vi "600 rpm peristaltic pump multiple heads (mLpermin).vi"(4 "State":i16, 5 "Time":dbl format="%.2f", 6 "Sensor Values":dbl[](array[numeric]), 7 "Set Points":dbl[](array[numeric])) -> (0 "required data":T1={"Set Point names"=["flow rate (mL/min)", "Tubing size code", "# of pump heads"], "required number of setpoints"=3, "required number of sensors"=0, "Sensor names"=[]}, 3 "output value":dbl)   [LabVIEW 2012]
panel:
  in  "pumpflow":dbl[unit][](array[numeric])=[9.549296547316535e-09, 3.342253804929783e-08, 1.2732395447351617e-07, 2.705634032562094e-07, 4.4563384065730255e-07, 6.04788783748884e-07] format="%.3f"
  in  "tubing size":enum16{"13", "14", "16", "25", "17", "18"}(ring)
  # "Enter the correct information for this control code in the required data structure below. Then make the current value default by right clicking on the border of the data structure."
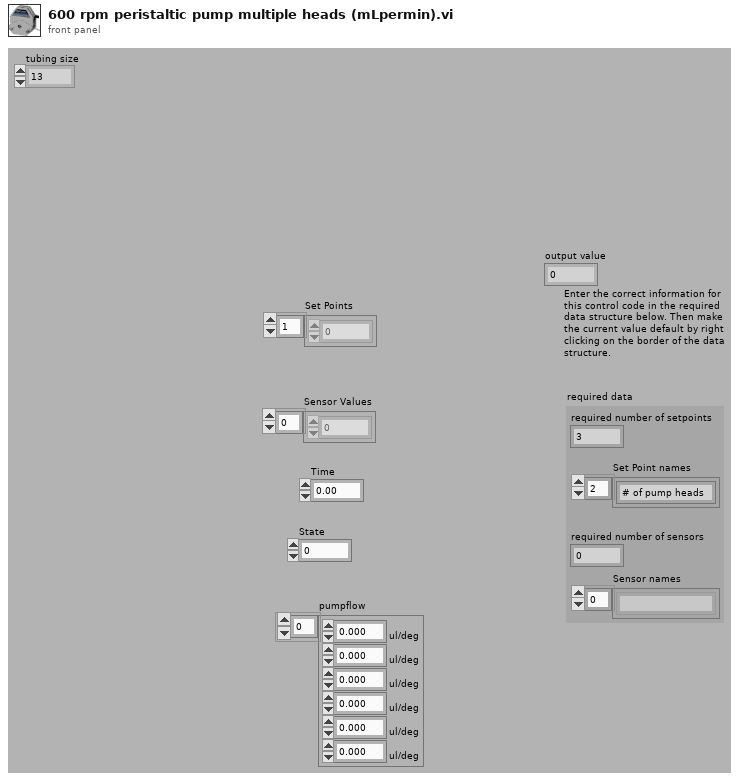
[diagram p1: front panel]
types:
  T1 = cluster{"Set Point names":string[], "required number of setpoints":u8, "required number of sensors":u8, "Sensor names":string[]}
  T2 = cluster{"Set Points[0]":dbl, "Set Points[1]":dbl, "Set Points[2]":dbl}
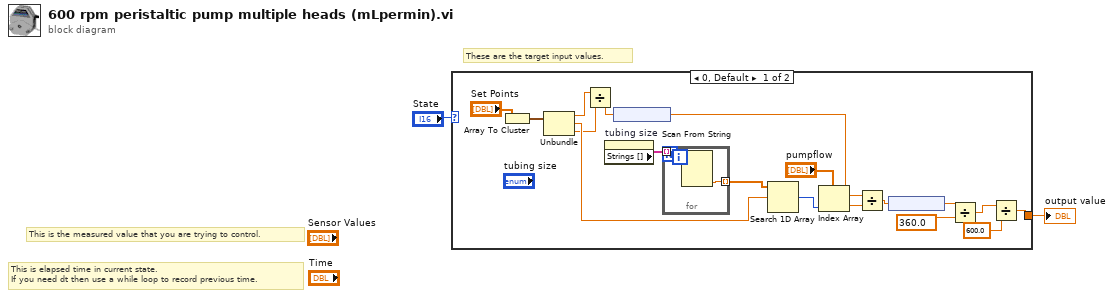
[diagram p0: block diagram]
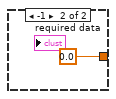
[diagram p2: hidden frame]
diagram:
  # "These are the target input values."
  # "This is the measured value that you are trying to control."
  # "This is elapsed time in current state.\nIf you need dt then use a while loop to record previous time."
  n1 = case shown="0, Default" "State" {
    tunnel: [w16 0.0 ("fraction on")] -> w1
    frame 0, Default {
      n2 = Array To Cluster(array="Set Points") -> (cluster=w20:T2)
      n3 = Unbundle(w20) -> ("Set Points[0]"=w7:dbl, "Set Points[1]"=w8:dbl, "Set Points[2]"=w6:dbl)
      n4 = Divide(x=w7, y=w6) -> (x/y=w5:dbl)
      n5 = property on="tubing size" class="Enum (strict)"() -> ("Strings []"=w17:string[])  [unwired: 2 in, 2 out]
      n6 = node(w5) -> (w9:dbl[unit])
      n7 = for {
        tunnel: w17 -> [w22] mode=indexing
        tunnel: [w21] -> w19 mode=indexing
        n8 = Scan From String(input string=w22) -> (output 1=w21:dbl)  [unwired: 4 in, 3 out]
      }
      n9 = Search 1D Array(1D array=w19, element=w8) -> (index of element=w10:i32)  [unwired: 1 in]
      n10 = Index Array(array="pumpflow", index=w10) -> (element=w14:dbl[unit])
      n11 = Divide(x=w9, y=w14) -> (x/y=w13:dbl[unit])
      n12 = node(w13) -> (w12:dbl)
      n13 = Divide(x=w12, y=360.0) -> (x/y=w4:dbl)
      n14 = Divide(x=w4, y=600.0 ("x")) -> (x/y=w16:dbl)
    }
    frame -1 {
    }
  }
  "output value" <- w1
